vi "exit_attempt1.vi"() -> ()   [LabVIEW 2015]
panel:
  in  "Tab Control":enum32{"Page 1", "Page 2", "Page 3"}(tab)
  in  "Next":bool
  in  "Close":bool
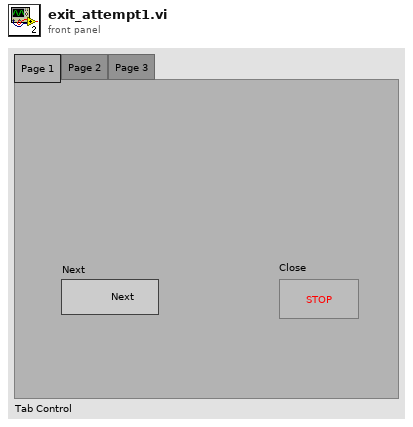
[diagram p1: front panel]
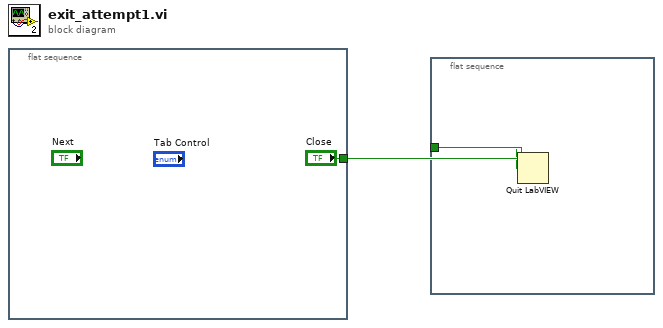
[diagram p0: block diagram]
diagram:
  n1 = flat-sequence {
    tunnel: ["Close"] -> w1
    frame #0 {
    }
  }
  n2 = flat-sequence {
    tunnel: w1 -> [w3]
    frame #0 {
      n3 = Quit LabVIEW(quit? (T)=w3) -> ()
    }
  }
